vi "Read Pressure.vi"(2 "error in (no error)":errorcluster, 3 "Max Pressure":dbl, 4 "AIDeviceRef":T1) -> (0 "Current Pressure":dbl)   [LabVIEW 2013]
uses:
  <vilib>/Rock Robotics/WPI/AnalogChannel/WPI_AnalogChannelDevRef.ctl
  <vilib>/Rock Robotics/SystemInterfaces/Typedef/FPGA_TypedefAnalogModule.ctl
  <vilib>/Rock Robotics/SystemInterfaces/AI/FPGA_AIChannel.ctl
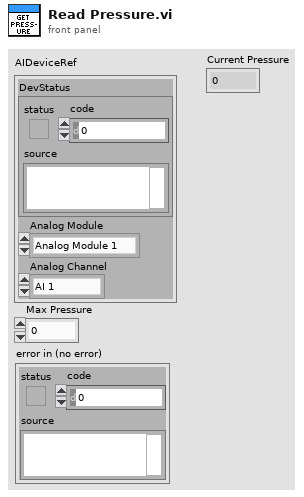
[diagram p1: front panel]
types:
  T1 = typedef "WPI_AnalogChannelDevRef.ctl" = cluster{"DevStatus":errorcluster, "Analog Module":T2, "Analog Channel":T3}
  T2 = typedef "FPGA_TypedefAnalogModule.ctl" = enum16{"Analog Module 1", "Analog Module 2"}
  T3 = typedef "FPGA_AIChannel.ctl" = enum8{"AI 1", "AI 2", "AI 3", "AI 4", "AI 5", "AI 6", "AI 7", "AI 8", "Invalid"}
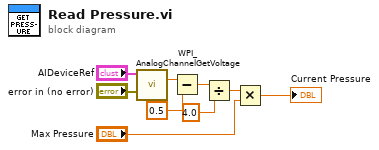
[diagram p0: block diagram]
diagram:
  n1 = call <vilib>:"WPI_AnalogChannelGetVoltage.vi"("error in (no error)"="error in (no error)", "AIDeviceRef"="AIDeviceRef") -> ("Voltage"=w7:dbl)  [unwired: 7 in, 2 out]
  n2 = Subtract(x=w7, y=0.5) -> (x-y=w5:dbl)
  n3 = Divide(x=w5, y=4.0) -> (x/y=w3:dbl)
  n4 = Multiply(x=w3, y="Max Pressure") -> (x*y=→"Current Pressure":dbl)
